vi "Test Black Levels.vi"(11 "Test Case In":refnum<class "Test.Camera.lvclass">) -> (0 "error out":errorcluster, 3 "Test Case Out":refnum<class "Test.Camera.lvclass">)   [LabVIEW 2020, in "Test.Camera.lvclass"]
uses:
  Test.Camera.lvclass
  C:/Program Files (x86)/National Instruments/LabVIEW 2020/vi.lib/Astemes/LUnit/Test Case.lvclass
  g_industrial_cam/Camera/Camera.lvclass/Camera.ctl
  <vilib>/Astemes/LUnit/Test Case.lvclass/Test Case.ctl
  g_industrial_cam/Camera/Auto Mode.ctl
  c3e2611f-c54f-4219-a549-b8da21c7f085.vi
  31b001b7-86ee-4e7d-b317-6e0f5f4be2a5.vi
  0aa1576c-e916-4ad0-9a97-64bd3e4eb69b.vi
  0aad262e-7ed0-45a2-a8a8-802ca94d5071.vi
  759e5037-5df0-4144-95b6-409846063909.vi
  g_industrial_cam/Camera/GetSetFrameRate.vi
  <vilib>/Astemes/LUnit/Append Pass Result.vi
  <vilib>/Astemes/LUnit/Append Fail Result.vi
  g_industrial_cam/Camera/GetSetBlackLevel.vi
  <vilib>/Astemes/LUnit/Describe Comparison.vi
  0aa1576c-e916-4ad0-9a97-64bd3e4eb69b.vi/9c5d11cd-9439-4240-a1ee-d9baace9c924.vi
  g_industrial_cam/Camera/GetSetBlackLevelAuto.vi
  759e5037-5df0-4144-95b6-409846063909.vi/9c5d11cd-9439-4240-a1ee-d9baace9c924.vi
  <vilib>/Astemes/LUnit/Run In UI.vi
  <vilib>/Utility/error.llb/Clear Errors.vi
  g_industrial_cam/Camera/Check Not Disconnected.vi
  <vilib>/Utility/error.llb/Error Cluster From Error Code.vi
  <vilib>/Astemes/LUnit/Describe Variant.vi
  <vilib>/Astemes/LUnit/Test Case.lvclass
  g_industrial_cam/Camera/Camera.lvclass
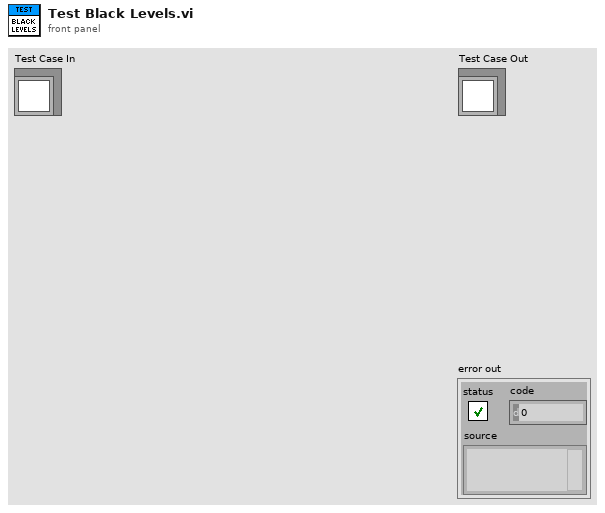
[diagram p1: front panel]
types:
  T1 = enum16{"Get Values", "Set Black Levels", "Enable Auto Black Level"}
  T2 = typedef "Camera.lvclass/Auto Mode.ctl" = enum8{"Off", "Once", "Continuous"}
  T3 = enum16{"Get Values", "Set Black Levels", "Enable Auto Black Level"}[]
  T4 = cluster{"Auto Avaliable":bool, "Min":dbl, "Max":dbl, "Black Level":dbl, "Avaliable":bool}
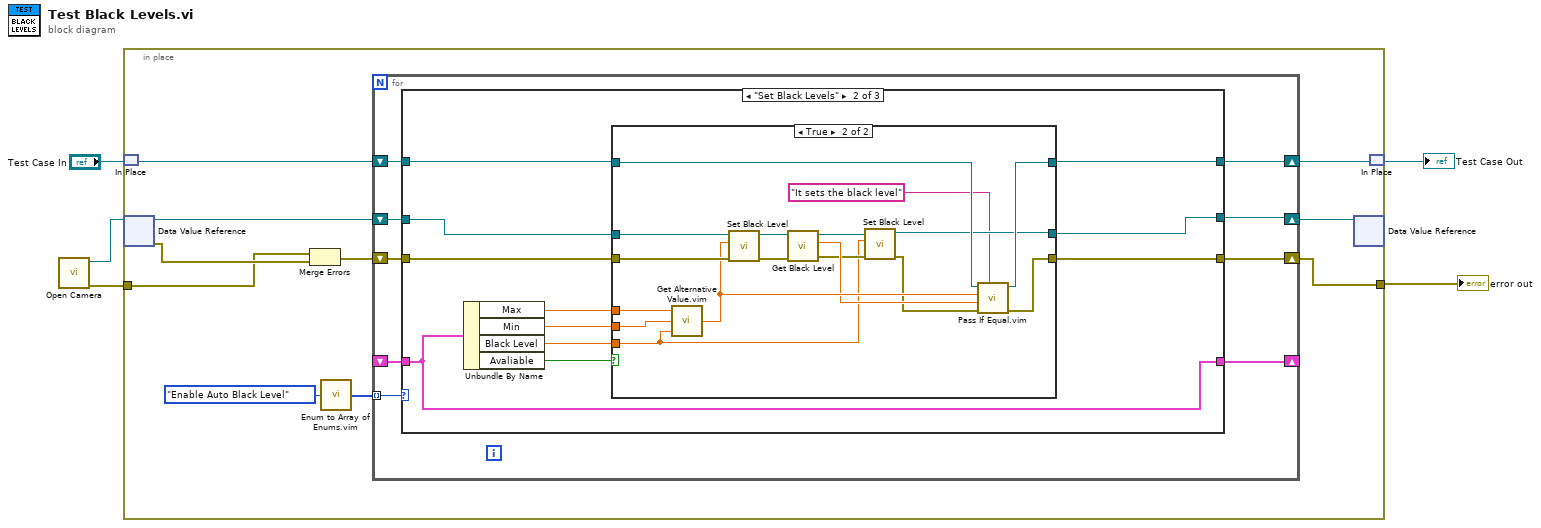
[diagram p0: block diagram]
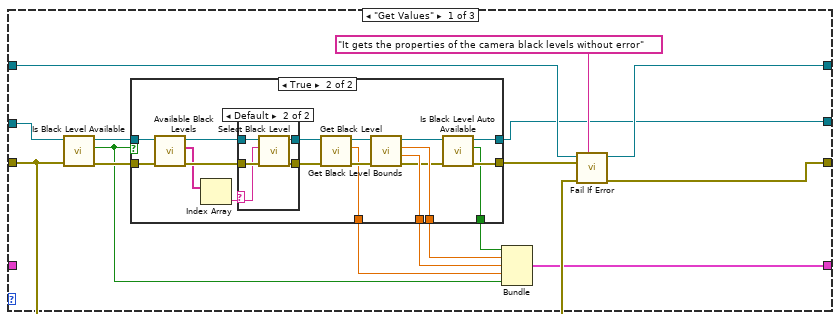
[diagram p2: hidden frame]
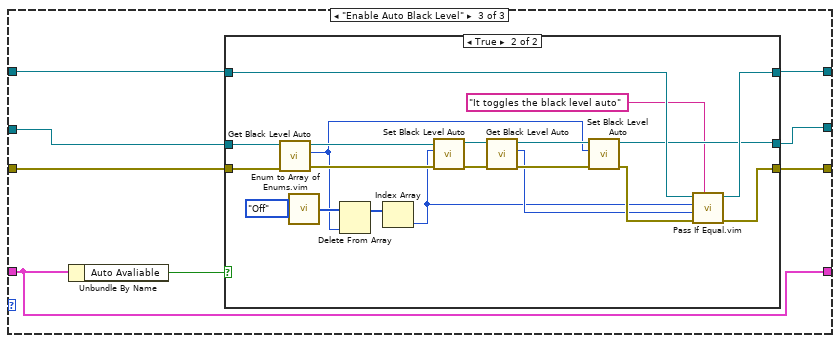
[diagram p6: hidden frame]
diagram:
  n1 = call "Open Camera.vi"() -> ("error out"=w5:errorcluster, "Camera"=w4:refnum<data-value>)  [unwired: 10 in]
  n2 = in-place {
    in-place-border: w5 -> [w8]
    in-place-border: [w7] -> w2
    n3 = in-place-match #1("Test Case In") -> (w10:refnum<class "Test.Camera.lvclass">)
    n4 = in-place-dvr #2(w4) -> (w14:refnum<class "Camera.lvclass">, w15:errorcluster)
    n5 = Merge Errors(w8, w15) -> (w13:errorcluster)
    n6 = call "Enum to Array of Enums.vim"("enum"=T1."Enable Auto Black Level") -> ("array of enums"=w11:T3)
    n7 = for {
      tunnel: w11 -> [w22] mode=indexing
      shift-right: [w21] -> w9
      shift-left: w14 -> [w24]
      shift-right: [w20] -> _
      shift-left: _ -> [w19]
      shift-right: [w17] -> w6
      shift-left: w10 -> [w18]
      shift-right: [w16] -> w7
      shift-left: w13 -> [w23]
      n8 = case shown="\"Set Black Levels\"" w22 {
        tunnel: w24 -> [w36 w77 w105]
        tunnel: w23 -> [w35 w78 w106]
        tunnel: [w28 w71 w102] -> w21
        tunnel: [w25 w69 w100] -> w20
        tunnel: w19 -> [_ w69 w100]
        tunnel: w18 -> [w40 w73 w104]
        tunnel: [w39 w72 w103] -> w17
        tunnel: [w37 w70 w101] -> w16
        frame "Get Values" {
          n9 = call "Is Black Level Available.vi"("error in (no error)"=w35, "Camera in"=w36) -> ("error out"=w34:errorcluster, "Avaliable"=w33:bool, "Camera"=w32:refnum<class "Camera.lvclass">)  [unwired: 7 in]
          n10 = case shown="True" w33 {
            tunnel: w34 -> [w41 w60]
            tunnel: w32 -> [w42 w50]
            tunnel: [_ w57] -> w31
            tunnel: [_ w55] -> w30
            tunnel: [w41 w53] -> w29
            tunnel: [w42 w56] -> w28
            tunnel: [_ w52] -> w27
            tunnel: [_ w43] -> w26
            frame False {
            }
            frame True {
              n11 = call "Available Black Levels.vi"("error in (no error)"=w60, "Camera in"=w50) -> ("error out"=w51:errorcluster, "Available Black Levels"=w48:string[], "Camera"=w49:refnum<class "Camera.lvclass">)  [unwired: 7 in]
              n12 = Index Array(array=w48) -> (element=w47:string)  [unwired: 1 in]
              n13 = case shown="Default" w47 {
                selector: w47 -> [_ w64]
                tunnel: [w61 w67] -> w59
                tunnel: w51 -> [w61 w66]
                tunnel: w49 -> [w62 w65]
                tunnel: [w62 w63] -> w45
                frame "" {
                }
                frame Default {
                  n14 = call "Select Black Level.vi"("error in (no error)"=w66, "Black Level Selection"=w64, "Camera in"=w65) -> ("error out"=w67:errorcluster, "Camera"=w63:refnum<class "Camera.lvclass">)  [unwired: 7 in]
                }
              }
              n15 = call "Get Black Level.vi"("error in (no error)"=w59, "Camera in"=w45) -> ("error out"=w46:errorcluster, "Black Level"=w43:dbl, "Camera"=w44:refnum<class "Camera.lvclass">)  [unwired: 7 in]
              n16 = call "Get Black Level Bounds.vi"("error in (no error)"=w46, "Camera in"=w44) -> ("error out"=w54:errorcluster, "Max"=w57:dbl, "Min"=w55:dbl, "Camera"=w58:refnum<class "Camera.lvclass">)  [unwired: 6 in]
              n17 = call "Is Black Level Auto Available.vi"("error in (no error)"=w54, "Camera in"=w58) -> ("error out"=w53:errorcluster, "Auto Avaliable"=w52:bool, "Camera"=w56:refnum<class "Camera.lvclass">)  [unwired: 7 in]
            }
          }
          n18 = Bundle("Auto Avaliable"=w27, "Min"=w30, "Max"=w31, "Black Level"=w26, "Avaliable"=w33) -> (w25:T4)  [unwired: 1 in]
          n19 = call <vilib>:"Fail If Error.vi"("Description"="It gets the properties of the camera black levels without error", "error in (no error)"=w35, "Assert error"=w29, "LUnit Test Case In"=w40) -> ("error out"=w37:errorcluster, "LUnit Test Case Out"=w39:refnum<class "Test.Camera.lvclass">)  [unwired: 6 in]
        }
        frame "Set Black Levels" {
          n20 = Unbundle By Name(w69) -> ("Max"=w76:dbl, "Min"=w75:dbl, "Black Level"=w74:dbl, "Avaliable"=w68:bool)
          n21 = case shown="True" w68 {
            tunnel: w78 -> [w81 w93]
            tunnel: w77 -> [w80 w92]
            tunnel: w76 -> [_ w98]
            tunnel: w75 -> [_ w97]
            tunnel: w74 -> [_ w82]
            tunnel: w73 -> [w79 w94]
            tunnel: [w79 w95] -> w72
            tunnel: [w80 w84] -> w71
            tunnel: [w81 w96] -> w70
            frame False {
            }
            frame True {
              n22 = call "Get Alternative Value.vim"("Value"=w82, "Min"=w97, "Max"=w98) -> ("Alternative Value"=w91:dbl)  [unwired: 1 in]
              n23 = call "Set Black Level.vi"("error in (no error)"=w93, "Black Level"=w91, "Camera in"=w92) -> ("error out"=w90:errorcluster, "Camera"=w89:refnum<class "Camera.lvclass">)  [unwired: 7 in]
              n24 = call "Get Black Level.vi"("error in (no error)"=w90, "Camera in"=w89) -> ("error out"=w87:errorcluster, "Black Level"=w88:dbl, "Camera"=w86:refnum<class "Camera.lvclass">)  [unwired: 7 in]
              n25 = call "Set Black Level.vi"("error in (no error)"=w87, "Black Level"=w82, "Camera in"=w86) -> ("error out"=w85:errorcluster, "Camera"=w84:refnum<class "Camera.lvclass">)  [unwired: 7 in]
              n26 = call "Pass If Equal.vim"("Description"="It sets the black level", "error in (no error)"=w85, "Actual"=w88, "Expected"=w91, "LUnit Test Case In"=w94) -> ("error out"=w96:errorcluster, "LUnit Test Case Out"=w95:refnum<class "Test.Camera.lvclass">)  [unwired: 5 in]
            }
          }
        }
        frame "Enable Auto Black Level" {
          n27 = Unbundle By Name(w100) -> ("Auto Avaliable"=w99:bool)
          n28 = case shown="True" w99 {
            tunnel: w106 -> [w109 w126]
            tunnel: w105 -> [w108 w125]
            tunnel: w104 -> [w107 w127]
            tunnel: [w107 w128] -> w103
            tunnel: [w108 w122] -> w102
            tunnel: [w109 w129] -> w101
            frame False {
            }
            frame True {
              n29 = call "Get Black Level Auto.vi"("error in (no error)"=w126, "Camera in"=w125) -> ("error out"=w124:errorcluster, "Auto Mode"=w112:T2, "Camera"=w119:refnum<class "Camera.lvclass">)  [unwired: 7 in]
              n30 = call "Enum to Array of Enums.vim"("enum"=Auto_Mode."Off" ("Auto Mode")) -> ("array of enums"=w114:T2[])
              n31 = Delete From Array(array=w114, index=w112) -> (array with subset deleted=w113:T2[])  [unwired: 1 in, 1 out]
              n32 = Index Array(array=w113) -> (element=w110:T2)  [unwired: 1 in]
              n33 = call "Set Black Level Auto.vi"("error in (no error)"=w124, "Mode"=w110, "Camera in"=w119) -> ("error out"=w120:errorcluster, "Camera"=w117:refnum<class "Camera.lvclass">)  [unwired: 7 in]
              n34 = call "Get Black Level Auto.vi"("error in (no error)"=w120, "Camera in"=w117) -> ("error out"=w118:errorcluster, "Auto Mode"=w111:T2, "Camera"=w116:refnum<class "Camera.lvclass">)  [unwired: 7 in]
              n35 = call "Set Black Level Auto.vi"("error in (no error)"=w118, "Mode"=w112, "Camera in"=w116) -> ("error out"=w123:errorcluster, "Camera"=w122:refnum<class "Camera.lvclass">)  [unwired: 7 in]
              n36 = call "Pass If Equal.vim"("Description"="It toggles the black level auto", "error in (no error)"=w123, "Actual"=w111, "Expected"=w110, "LUnit Test Case In"=w127) -> ("error out"=w129:errorcluster, "LUnit Test Case Out"=w128:refnum<class "Test.Camera.lvclass">)  [unwired: 5 in]
            }
          }
        }
      }
    }
    n37 = in-place-dvr #2(w9) -> ()  [unwired: 2 out]
    n38 = in-place-match #1(w6) -> (→"Test Case Out":refnum<class "Test.Camera.lvclass">)
  }
  "error out" <- w2
